vi "Switch Subpanel.vi"(8 "error in (no error)":errorcluster, 9 "Calling VI":refnum<vi>, 10 "Subpanel Type":T1, 11 "CIF_UI in":refnum<class "CIF_UI.lvclass">) -> (0 "error out":errorcluster, 2 "VI Reference":refnum<vi>, 3 "CIF_UI out":refnum<class "CIF_UI.lvclass">)   [LabVIEW 2021, in "CIF_UI.lvclass"]
uses:
  CIF_UI.lvclass
  Typedef/Subpanel Type.ctl
  CIF_UI.lvclass/CIF_UI.ctl
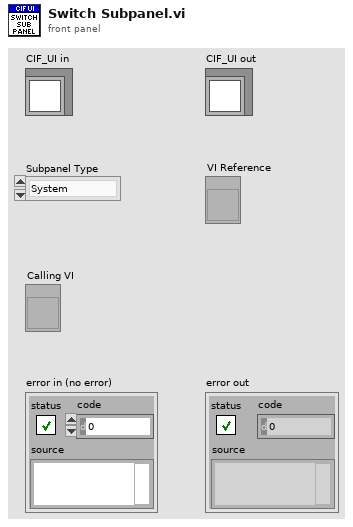
[diagram p1: front panel]
types:
  T1 = typedef "CIF_UI.lvclass/Subpanel Type.ctl" = enum16{"System", "Errors", "Channel", "Plugin"}
  T2 = typedef "CIF_UI.lvclass/Subpanel Map.ctl" = map{T1, T3}
  T3 = typedef "CIF_UI.lvclass/Subpanel Data.ctl" = cluster{"VI Reference":refnum<vi>, "Plugin Subpanel Events":T4}
  T4 = typedef "CIF_UI.lvclass/Plugin Subpanel Events.ctl" = cluster{"Plugin Shutdown":refnum<user-event>}
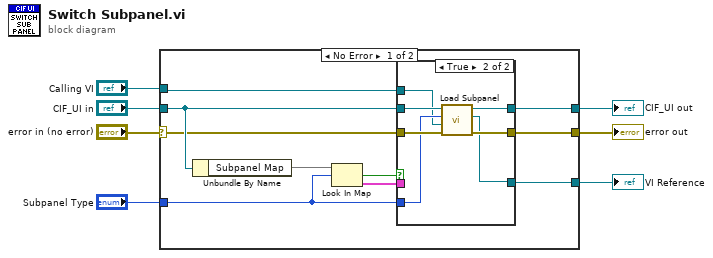
[diagram p0: block diagram]
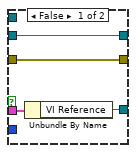
[diagram p2: hidden frame]
diagram:
  n1 = case shown="No Error" "error in (no error)" {
    selector: "error in (no error)" -> [w11 w30]
    tunnel: [w10 w30] -> w6
    tunnel: [w12 w29] -> w4
    tunnel: "CIF_UI in" -> [w14 w29]
    tunnel: "Subpanel Type" -> [w13 _]
    tunnel: [w9 _] -> w2
    tunnel: "Calling VI" -> [w8 _]
    frame No Error {
      n2 = Unbundle By Name(w14) -> ("Subpanel Map"=w17:T2)
      n3 = Look In Map(map=w17, key=w13) -> (key not found?=w16:bool, value=w15:T3)  [unwired: 1 in]
      n4 = case shown="True" w16 {
        tunnel: w15 -> [w21 _]
        tunnel: w14 -> [w20 w28]
        tunnel: w13 -> [_ w25]
        tunnel: [w20 w27] -> w12
        tunnel: w11 -> [w19 w26]
        tunnel: [w19 w24] -> w10
        tunnel: [w18 w23] -> w9
        tunnel: w8 -> [_ w22]
        frame False {
          n5 = Unbundle By Name(w21) -> ("VI Reference"=w18:refnum<vi>)
        }
        frame True {
          n6 = call "Load Subpanel.vi"("error in (no error)"=w26, "Calling VI"=w22, "Subpanel Type"=w25, "CIF_UI in"=w28) -> ("error out"=w24:errorcluster, "VI Reference"=w23:refnum<vi>, "CIF_UI out"=w27:refnum<class "CIF_UI.lvclass">)  [unwired: 5 in]
        }
      }
    }
    frame Error {
    }
  }
  "error out" <- w6
  "CIF_UI out" <- w4
  "VI Reference" <- w2
